vi "SQLite Edit Category Test.vi"(8 "Error In (no error)":errorcluster, 11 "DB Operator In":refnum<class "DB Operator.lvclass">) -> (0 "Error Out":errorcluster, 3 "DB Operator Out":refnum<class "DB Operator.lvclass">)   [LabVIEW 2023]
uses:
  DB Operator/DB Operator.lvclass
  SQLite DB Operator/SQLite DB Operator.lvclass
  H:/Desktop/LabVIEW/LabView Repo/Expenses-Tracker-DB-Operator/DB Operator/DB Operator.lvclass
  DB Operator/Public/Ctrls/DB Controls/Category.ctl
  SQLite DB Operator/SQLite DB Operator.lvclass/SQLite DB Operator.ctl
  <vilib>/drjdpowell/SQLite Library/SQL Connection/Execute SQL (No results).vi
  <vilib>/drjdpowell/SQLite Library/SQL Connection/Execute SQL (Variant Cluster results).vi
  <vilib>/addons/_JKI Toolkits/Caraya/classes/Assert/Assert Equal Value_Variant.vi
  <vilib>/addons/_JKI Toolkits/Caraya/classes/Assert/Assert Not Equal Value_Variant.vi
  <vilib>/drjdpowell/SQLite Library/SQL Connection/Connection.lvclass
  <vilib>/addons/_JKI Toolkits/Caraya/classes/Test/Test.lvclass
  <vilib>/drjdpowell/SQLite Library/SQLite.lvlib
  <vilib>/addons/_JKI Toolkits/Caraya/classes/Assert/Assert.lvclass
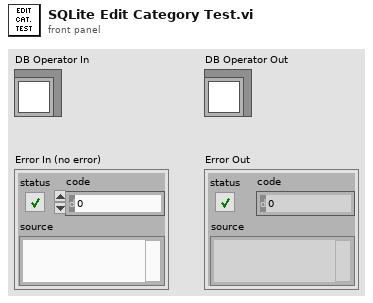
[diagram p1: front panel]
types:
  T1 = typedef "DB Operator.lvclass/Category.ctl" = cluster{"ID":u32, "Name":string}
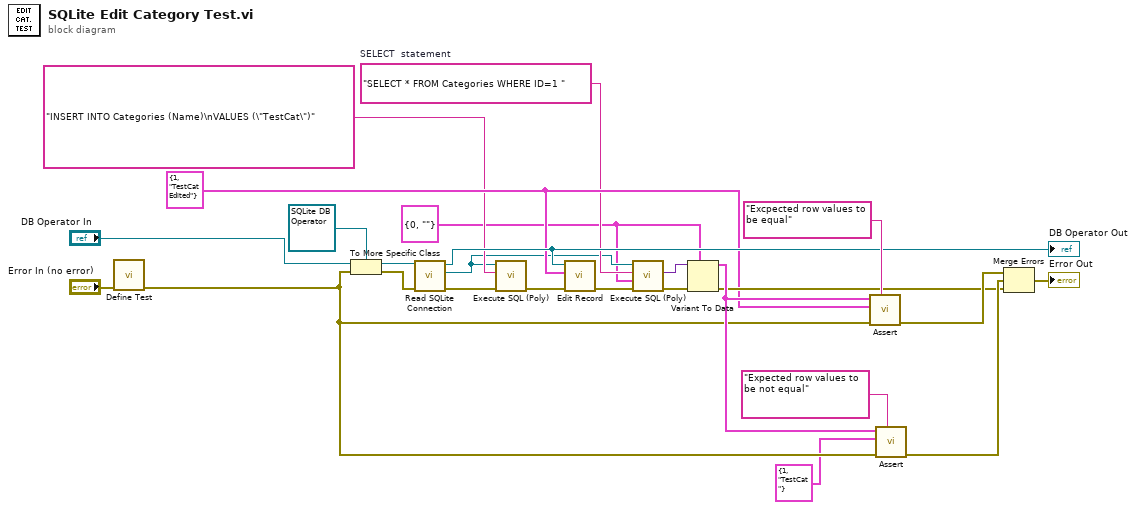
[diagram p0: block diagram]
diagram:
  w2 = T1 {"ID"=0, "Name"=""} ("Category")
  w9 = T1 {"ID"=1, "Name"="TestCatEdited"} ("Category")
  w6 = "SELECT * FROM Categories WHERE ID=1 "  # SELECT  statement
  n1 = call <vilib>:"Define Test.vi"("error in (no error)"="Error In (no error)") -> ("error out"=w13:errorcluster)  [unwired: 9 in, 1 out]
  n2 = To More Specific Class(target class=refnum<class "SQLite DB Operator.lvclass"> refnum ("SQLite DB Operator.lvclass"), reference="DB Operator In", error in=w13) -> (specific class reference=w25:refnum<class "SQLite DB Operator.lvclass">, error out=w19:errorcluster)
  n3 = call "Read SQLite Connection.vi"("Error In (no error)"=w19, "SQLite DB Operator In"=w25) -> ("Error Out"=w23:errorcluster, "SQLite.lvlib:Connection"=w5:refnum<class "Connection.lvclass">, "SQLite DB Operator out"=w10:refnum<class "SQLite DB Operator.lvclass">)  [unwired: 7 in]
  "DB Operator Out" <- w10
  n4 = call-poly <vilib>:"Execute SQL (Poly).vi"("error in (no error)"=w23, "SQL"="INSERT INTO Categories (Name)\nVALUES (\"TestCat\")", "SQLite Connection in"=w5) -> ("error out"=w11:errorcluster)  [unwired: 7 in, 1 out]
  n5 = call-dynamic "Edit Record.vi"("Error In (no error)"=w11, "Data"=w9, "DB Operator in"=w10) -> ("Error Out"=w7:errorcluster)  [unwired: 7 in, 1 out]
  n6 = call-poly <vilib>:"Execute SQL (Poly).vi"("error in (no error)"=w7, "Cluster"=w2, "SQL"=w6, "SQLite Connection in"=w5) -> ("error out"=w3:errorcluster, "Result (use Variant to Data)"=w4:variant)  [unwired: 5 in, 1 out]
  n7 = Variant To Data(error in=w3, type=w2, Variant=w4) -> (data=w17:T1, error out=w14:errorcluster)
  n8 = call-poly <vilib>:"Assert.vi"("Label"="Excpected row values to be equal" ("Label (VI Title)"), "error in (no error)"=w13, "Y"=w9, "X"=w17) -> ("error out"=w20:errorcluster)  [unwired: 6 in, 1 out]
  n9 = call-poly <vilib>:"Assert.vi"("Label"="Expected row values to be not equal" ("Label (VI Title)"), "error in (no error)"=w13, "Y"=T1 {"ID"=1, "Name"="TestCat"} ("Category"), "X"=w17) -> ("error out"=w15:errorcluster)  [unwired: 6 in, 1 out]
  n10 = Merge Errors(w20, w15, w14) -> (→"Error Out":errorcluster)
